vi "CRYEmpty One Data.vi"(9 "Index":i32[](array[numeric]), 10 "sOption":string, 11 "Type":enum16{"Curves", "Values", "Results", "WFM"}(ring)) -> ()   [LabVIEW 2013]
uses:
  CRYSystem/Task Sequence/CRYProject Run Control Global.vi
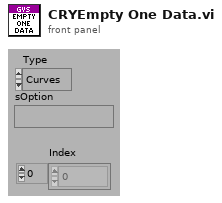
[diagram p1: front panel]
types:
  T1 = typedef "CRYData Cluster.ctl" = cluster{"Name":string, "Curve":cluster{"x":dbl, "y":dbl, "z":dbl}[], "X data":u16, "Y data":u16, "Z data":u16, "X axis":u16, "Y axis":u16, "Z axis":u16, "X unit":string, "Y unit":string, "Z unit":string, "X dB ref":dbl, "Y dB ref":dbl, "Z dB ref":dbl, "single val":bool, "protected":bool, "display X":bool, "display Y":bool, "display Z":bool, "Test Info":string, "Step No.":i32, "Plot Settings":cluster{"Color":u32, "Interpolation":u8, "Point Style":u8, "Line Style":u8, "Point Color":u32, "Line Width":u8, "Bar Plot Style":u8, "Fill To":i16}, "AutoProtect":bool}
  T2 = typedef "CRYWaveform Cluster.ctl" = cluster{"Waveform":cluster{"X0":dbl, "dX":dbl, "Y":sgl[]}, "X data":u16, "Y data":u16, "Y axis":u16, "X unit":string, "Y unit":string, "Y dB ref":dbl, "display Y":bool, "display X":bool, "Overload?":bool, "Test Info":string, "Step No.":i32, "Name":string, "protected":bool, "Sqc history":string[], "Signal Channel ID":i32, "Plot Settings":cluster{"Color":u32, "Interpolation":u8, "Point Style":u8, "Line Style":u8, "Point Color":u32, "Line Width":u8, "Bar Plot Style":u8, "Fill To":i16}, "AutoProtect":bool}
  T3 = typedef "CRYResult Cluster.ctl" = cluster{"Name":string, "Margin":dbl, "unit":string, "Verdict":bool, "Limit":string, "Max/Min":string, "protected":bool, "Step No.":i32, "Test Info":string, "AutoProtect":bool}
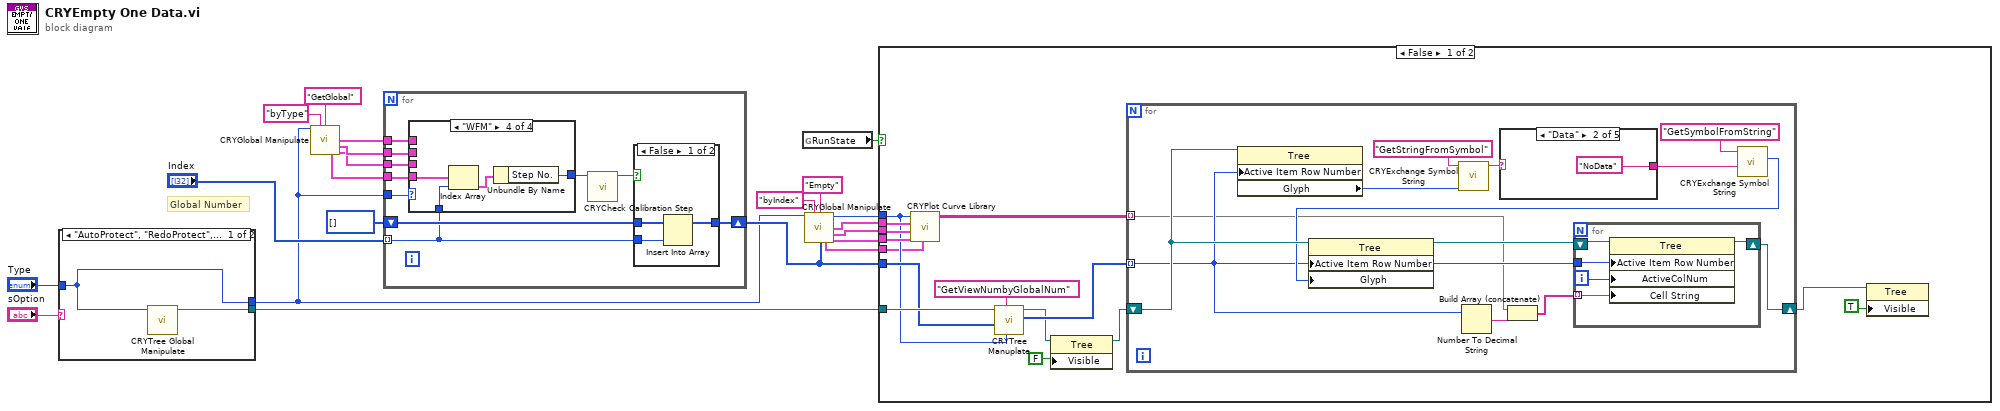
[diagram p0: block diagram]
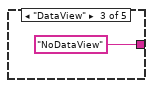
[diagram p3: hidden frame]
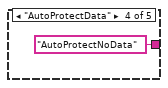
[diagram p4: hidden frame]
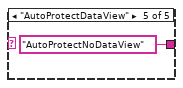
[diagram p5: hidden frame]
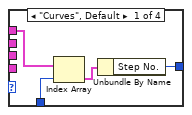
[diagram p8: hidden frame]
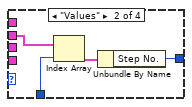
[diagram p9: hidden frame]
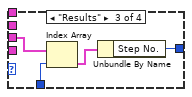
[diagram p10: hidden frame]
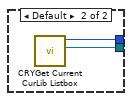
[diagram p11: hidden frame]
diagram:
  # "Global Number"
  n1 = case shown="\"AutoProtect\", \"RedoProtect\", \"Some\"" "sOption" {
    tunnel: [w23 w25] -> w7
    tunnel: [w22 w24] -> w8
    tunnel: "Type" -> [w23 _]
    frame "AutoProtect", "RedoProtect", "Some" {
      n2 = call "CRYTree Global Manipulate.vi"("Type In"=w23) -> ("Tree/Curve Tree"=w22:refnum<vi>)  [unwired: 7 in, 3 out]
    }
    frame Default {
      n3 = call "CRYGet Current CurLib Listbox.vi"() -> ("CurLib Tree"=w24:refnum<vi>, "Type"=w25:enum16{"Curves", "Values", "Results", "WFM"})  [unwired: 9 in, 1 out]
    }
  }
  n4 = call "CRYGlobal Manipulate.vi"("Type"=w7, "sOption"="byType", "sAction"="GetGlobal") -> ("Curves Out"=w6:T1[], "Values Out"=w5:T1[], "WFM Out"=w3:T2[], "Results Out"=w4:T3[])  [unwired: 6 in, 3 out]
  n5 = for {
    tunnel: w7 -> [w34]
    tunnel: "Index" -> [w30] mode=indexing
    shift-right: [w31] -> w12
    shift-left: i32[] [] ("Index") -> [w32]
    tunnel: w6 -> [w29]
    tunnel: w5 -> [w28]
    tunnel: w4 -> [w27]
    tunnel: w3 -> [w26]
    n6 = case shown="\"WFM\"" w34 {
      tunnel: [w43 w47 w51 w55] -> w35
      tunnel: w30 -> [w41 w45 w50 w54]
      tunnel: w29 -> [w40 _ _ _]
      tunnel: w28 -> [_ w44 _ _]
      tunnel: w27 -> [_ _ w48 _]
      tunnel: w26 -> [_ _ _ w52]
      frame "Curves", Default {
        n7 = Index Array(array=w40, index=w41) -> (element=w42:T1)
        n8 = Unbundle By Name(w42) -> ("Step No."=w43:i32)
      }
      frame "Values" {
        n9 = Index Array(array=w44, index=w45) -> (element=w46:T1)
        n10 = Unbundle By Name(w46) -> ("Step No."=w47:i32)
      }
      frame "Results" {
        n11 = Index Array(array=w48, index=w50) -> (element=w49:T3)
        n12 = Unbundle By Name(w49) -> ("Step No."=w51:i32)
      }
      frame "WFM" {
        n13 = Index Array(array=w52, index=w54) -> (element=w53:T2)
        n14 = Unbundle By Name(w53) -> ("Step No."=w55:i32)
      }
    }
    n15 = call "CRYCheck Calibration Step.vi"("Step No"=w35) -> ("Is Calibration?"=w33:bool)  [unwired: 9 in, 1 out]
    n16 = case shown="False" w33 {
      tunnel: w32 -> [w38 w39]
      tunnel: [w37 w39] -> w31
      tunnel: w30 -> [w36 _]
      frame False {
        n17 = Insert Into Array(array=w38, new element=w36) -> (w37:i32[])  [unwired: 1 in]
      }
      frame True {
      }
    }
  }
  n18 = global read "CRYProject Run Control Global.vi" "RunState"() -> (w17:bool)
  n19 = call "CRYGlobal Manipulate.vi"("Type"=w7, "sOption"="byIndex", "sAction"="Empty", "nData"=w12) -> ("Type out"=w14:enum16{"Curves", "Values", "Results", "WFM"}, "Curves Out"=w13:T1[], "Values Out"=w16:T1[], "WFM Out"=w1:T2[], "Results Out"=w15:T3[])  [unwired: 5 in, 2 out]
  n20 = case shown="False" w17 {
    tunnel: w8 -> [w65 _]
    tunnel: w16 -> [w68 _]
    tunnel: w15 -> [w67 _]
    tunnel: w12 -> [w64 _]
    tunnel: w14 -> [w62 _]
    tunnel: w13 -> [w69 _]
    tunnel: w1 -> [w61 _]
    frame False {
      n21 = call "CRYPlot Curve Library.vi"("Waveform"=w61, "Results"=w67, "Values"=w68, "Curves"=w69, "Type"=w62) -> ("PlotStrings"=w70:string[][])  [unwired: 6 in]
      n22 = call "CRYTree Manuplate.vi"("Type"=w62, "sAction"="GetViewNumbyGlobalNum", "nData"=w64, "Tree in"=w65) -> ("nData Out"=w63:i32[], "Tree Out"=w58:refnum<vi>)  [unwired: 4 in, 2 out]
      n23 = property class="Tree"(reference=w58, "Visible"=FALSE) -> (reference out=w57:refnum<vi>)  [unwired: 1 in, 1 out]
      n24 = for {
        tunnel: w70 -> [w72] mode=indexing
        tunnel: w63 -> [w75] mode=indexing
        shift-right: [w71] -> w56
        shift-left: w57 -> [w82]
        n25 = property on="Property Node" class="Tree"(reference=w82, "Active Item Row Number"=w75) -> ("Glyph"=w80:i32)  [unwired: 1 in, 2 out]
        n26 = call "CRYExchange Symbol String.vi"("nData"=w80, "sAction"="GetStringFromSymbol") -> ("sData out"=w78:string)  [unwired: 8 in, 1 out]
        n27 = Number To Decimal String(number=w75) -> (decimal integer string=w74:string)  [unwired: 1 in]
        n28 = case shown="\"Data\"" w78 {
          selector: w78 -> [w84 _ _ _ _]
          tunnel: [w84 "NoData" ("sData") "NoDataView" ("sData") "AutoProtectNoData" ("sData") "AutoProtectNoDataView" ("sData")] -> w77
          frame Default {
          }
          frame "Data" {
          }
          frame "DataView" {
          }
          frame "AutoProtectData" {
          }
          frame "AutoProtectDataView" {
          }
        }
        n29 = Build Array (concatenate)(w72, w74) -> (w73:string[])
        n30 = call "CRYExchange Symbol String.vi"("sData"=w77, "sAction"="GetSymbolFromString") -> ("nData out"=w76:i32)  [unwired: 8 in, 1 out]
        n31 = property on="Property Node" class="Tree"(reference=w82, "Active Item Row Number"=w75, "Glyph"=w76) -> (reference out=w83:refnum<vi>)  [unwired: 1 in, 1 out]
        n32 = for {
          shift-right: [w92] -> w71
          shift-left: w83 -> [w93]
          tunnel: w75 -> [w91]
          tunnel: w73 -> [w89] mode=indexing
          i -> [w90]
          n33 = property on="Property Node" class="Tree"(reference=w93, "Active Item Row Number"=w91, "ActiveColNum"=w90, "Cell String"=w89) -> (reference out=w92:refnum<vi>)  [unwired: 1 in, 1 out]
        }
      }
      n34 = property class="Tree"(reference=w56, "Visible"=TRUE) -> ()  [unwired: 1 in, 2 out]
    }
    frame True {
    }
  }
